vi "Bundle temperatures.vi"(9 "Sample":dbl, 10 "VTI space":dbl, 11 "LSC218 sensors":T1 {"Time stamp" format="%<%H:%M:%S%2u\n%Y/%m/%d>T"}) -> (3 "Tmp [K]":T2)   [LabVIEW 2024]
uses:
  Subsystem modules/Magnet module/ctl/Cryostat temperature sensors.ctl
  <vilib>/GPower/Numeric/Library/Average/AvrgDBL.vi
  <vilib>/GPower/Numeric/GPNumeric.lvlib
  Subsystem modules/Magnet module/Magnet module.lvlib
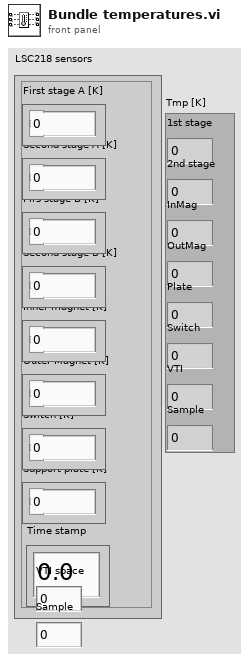
[diagram p1: front panel]
types:
  T1 = typedef "Magnet module.lvlib/Cryostat temperature sensors.ctl" = cluster{"First stage A [K]":dbl, "Second stage A [K]":dbl, "Firs stage B [K]":dbl, "Second stage B [K]":dbl, "Inner magnet [K]":dbl, "Outer Magnet [K]":dbl, "Switch [K]":dbl, "Support plate [K]":dbl, "Time stamp":dbl}
  T2 = cluster{"1st stage":dbl, "2nd stage":dbl, "InMag":dbl, "OutMag":dbl, "Plate":dbl, "Switch":dbl, "VTI":dbl, "Sample":dbl}
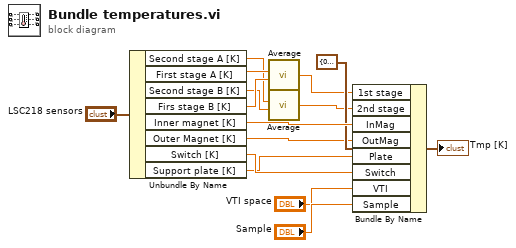
[diagram p0: block diagram]
diagram:
  n1 = Unbundle By Name("LSC218 sensors") -> ("Second stage A [K]"=w6:dbl, "First stage A [K]"=w9:dbl, "Second stage B [K]"=w7:dbl, "Firs stage B [K]"=w10:dbl, "Inner magnet [K]"=w15:dbl, "Outer Magnet [K]"=w1:dbl, "Switch [K]"=w3:dbl, "Support plate [K]"=w2:dbl)
  n2 = call-poly <vilib>:"Average.vi"("b"=w10, "a"=w9) -> ("Average of a and b"=w11:dbl)  [unwired: 4 in]
  n3 = call-poly <vilib>:"Average.vi"("b"=w7, "a"=w6) -> ("Average of a and b"=w8:dbl)  [unwired: 4 in]
  n4 = Bundle By Name(cluster=T2 {"1st stage"=0.0, "2nd stage"=0.0, "InMag"=0.0, "OutMag"=0.0, "Plate"=0.0, "Switch"=0.0, "VTI"=0.0, "Sample"=0.0} ("Tmp [K]"), "1st stage"=w11, "2nd stage"=w8, "InMag"=w15, "OutMag"=w1, "Plate"=w2, "Switch"=w3, "VTI"="VTI space", "Sample"="Sample") -> (→"Tmp [K]":T2)
